vi "Get Display Text.vi"(8 "error in (no error)":errorcluster, 11 "Attribute in":refnum<class "Attribute.lvclass">) -> (0 "error out":errorcluster, 1 "Detail Text":string, 2 "Display Name":string, 3 "Attribute out":refnum<class "Attribute.lvclass">)   [LabVIEW 2023, in "VILab.lvlib" / "Attribute.lvclass"]
uses:
  Attribute.lvclass
  Attribute.lvclass/Attribute.ctl
  Data Item/Data Item.lvclass
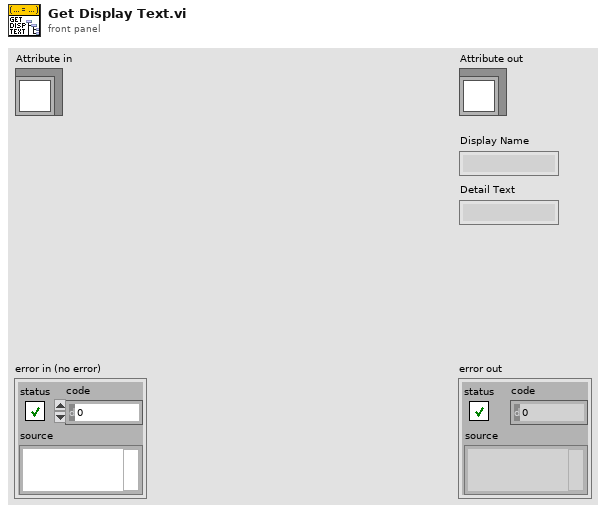
[diagram p1: front panel]
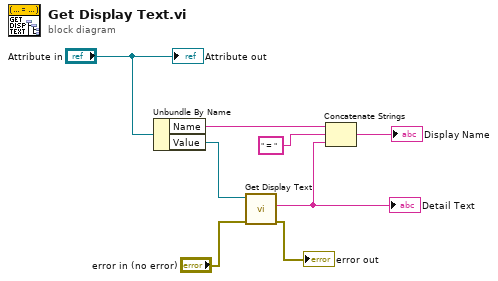
[diagram p0: block diagram]
diagram:
  n1 = Unbundle By Name("Attribute in") -> ("Name"=w4:string, "Value"=w7:refnum<class "Data Item.lvclass">)
  n2 = call-dynamic "Get Display Text.vi"("error in (no error)"="error in (no error)", "Data Item in"=w7) -> ("error out"=→"error out":errorcluster, "Display Name"=w3:string)  [unwired: 6 in, 2 out]
  "Detail Text" <- w3
  n3 = Concatenate Strings(w4, " = ", w3) -> (→"Display Name":string)
  "Attribute out" <- "Attribute in"
